vi "GetPathToClass.vi"(8 "error in (no error)":errorcluster, 10 "configuration file path":path=path "") -> (0 "error IO":errorcluster, 2 "PathToClass":path)   [LabVIEW 2014, in "NistBaseClasses.lvlib" / "NISTObject.lvclass"]
uses:
  NISTObject.lvclass
  <vilib>/Utility/config.llb/Read Key (Path).vi
  <vilib>/Utility/config.llb/NI_LVConfig.lvlib
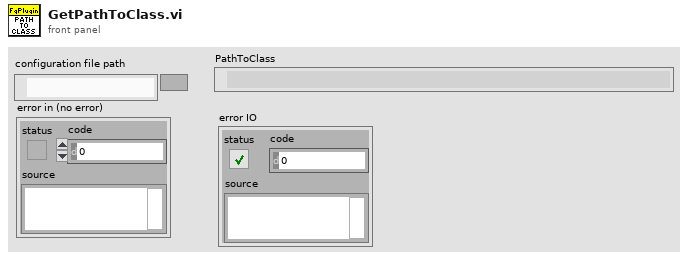
[diagram p1: front panel]
types:
  T1 = typedef "NI_LVConfig.lvlib/Config Data RefNum.ctl" = refnum<k1>
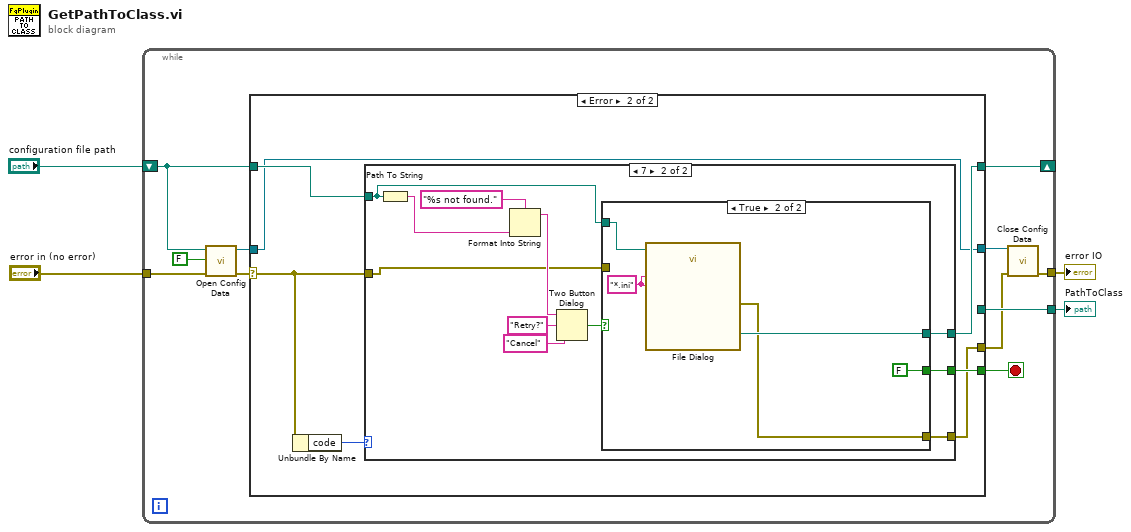
[diagram p0: block diagram]
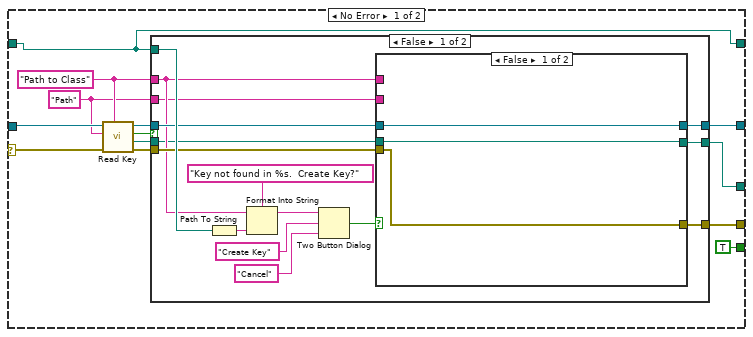
[diagram p2: hidden frame]
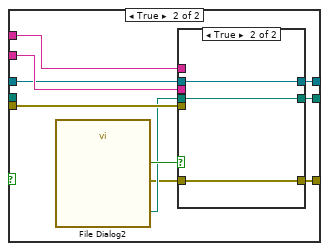
[diagram p3: hidden frame]
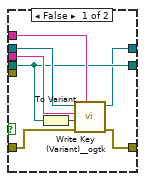
[diagram p4: hidden frame]
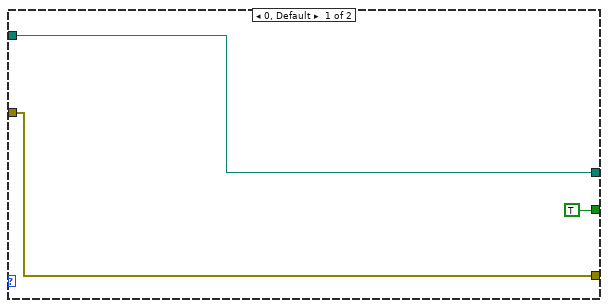
[diagram p6: hidden frame]
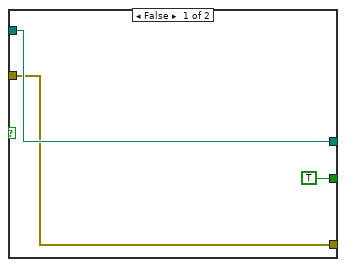
[diagram p7: hidden frame]
diagram:
  n1 = while {
    tunnel: "error in (no error)" -> [w15]
    shift-right: [w11] -> _
    shift-left: "configuration file path" -> [w5]
    tunnel: [w6] -> w2
    tunnel: [w9] -> w1
    stop <- w10 stop-if-true
    n2 = call <vilib>:"Open Config Data.vi"("error in (no error)"=w15, "create file if necessary (T)"=FALSE, "configuration file path"=w5) -> ("error out"=w13:errorcluster, "refnum"=w12:T1)  [unwired: 6 in, 1 out]
    n3 = case shown="Error" w13 {
      selector: w13 -> [w26 w73]
      tunnel: w12 -> [w27 w71]
      tunnel: w5 -> [w20 w76]
      tunnel: [w20 w75] -> w11
      tunnel: [TRUE w74] -> w10
      tunnel: [w17 w72] -> w7
      tunnel: [w18 _] -> w9
      tunnel: [w16 w71] -> w8
      frame No Error {
        w21 = "Path" ("key")
        w24 = "Path to Class" ("section")
        n4 = call-poly <vilib>:"Read Key.vi"("section"=w24, "error in (no error)"=w26, "key"=w21, "refnum"=w27) -> ("error out"=w23:errorcluster, "value"=w19:path, "found?"=w25:bool, "refnum out"=w22:T1)  [unwired: 4 in]
        n5 = case shown="False" w25 {
          tunnel: w24 -> [w34 _]
          tunnel: w23 -> [w36 w69]
          tunnel: w20 -> [w41 _]
          tunnel: w22 -> [w35 w68]
          tunnel: w21 -> [w33 _]
          tunnel: w19 -> [w32 w70]
          tunnel: [w31 w70] -> w18
          tunnel: [w30 w69] -> w17
          tunnel: [w29 w68] -> w16
          frame False {
            n6 = Path To String(path=w41) -> (string=w42:string)
            n7 = Format Into String(format string="Key not found in %s.  Create Key?", initial string=w34, w42) -> (resulting string=w40:string)  [unwired: 1 in, 1 out]
            n8 = Two Button Dialog(message=w40, 1:"Cancel" ("F button name (\"Cancel\")"), 2:"Create Key" ("T button name (\"OK\")")) -> (T button?=w37:bool)
            n9 = case shown="False" w37 {
              tunnel: w36 -> [w45 w54]
              tunnel: w35 -> [w44 w55]
              tunnel: w34 -> [_ w53]
              tunnel: w33 -> [_ w56]
              tunnel: w32 -> [w46 _]
              tunnel: [w46 w50] -> w31
              tunnel: [w45 w49] -> w30
              tunnel: [w44 w47] -> w29
              frame False {
              }
              frame True {
                n10 = call "File Dialog2"() -> ("selected path"=w51:path, "cancelled"=w52:bool, "error out"=w48:errorcluster)  [unwired: 12 in, 1 out]
                n11 = case shown="True" w52 {
                  tunnel: w56 -> [w64 _]
                  tunnel: w55 -> [w63 w65]
                  tunnel: w54 -> [_ _]
                  tunnel: w53 -> [w62 _]
                  tunnel: w51 -> [w60 w67]
                  tunnel: [w60 w67] -> w50
                  tunnel: [w58 w66] -> w49
                  tunnel: w48 -> [w59 w66]
                  tunnel: [w57 w65] -> w47
                  frame False {
                    n12 = To Variant(anything=w60) -> (Variant=w61:variant)
                    n13 = call <userlib>:"Write Key (Variant)__ogtk.vi"("section"=w62, "error in (no error)"=w59, "key-value"=w61, "key (optional)"=w64, "refnum"=w63) -> ("error out"=w58:errorcluster, "refnum out"=w57:T1)  [unwired: 5 in]
                  }
                  frame True {
                  }
                }
              }
            }
          }
          frame True {
          }
        }
      }
      frame Error {
        n14 = Unbundle By Name(w73) -> ("code"=w77:i32)
        n15 = case shown="7" w77 {
          tunnel: w76 -> [w78 w86]
          tunnel: [w78 w85] -> w75
          tunnel: [TRUE w84] -> w74
          tunnel: w73 -> [w79 w83]
          tunnel: [w79 w82] -> w72
          frame 0, Default {
          }
          frame 7 {
            n16 = Path To String(path=w86) -> (string=w81:string)
            n17 = Format Into String(format string="%s not found.", w81) -> (resulting string=w90:string)  [unwired: 2 in, 1 out]
            n18 = Two Button Dialog(message=w90, 1:"Cancel" ("F button name (\"Cancel\")"), 2:"Retry?" ("T button name (\"OK\")")) -> (T button?=w87:bool)
            n19 = case shown="True" w87 {
              tunnel: w86 -> [w93 w95]
              tunnel: [w93 w98] -> w85
              tunnel: [TRUE FALSE] -> w84
              tunnel: w83 -> [w92 _]
              tunnel: [w92 w96] -> w82
              frame False {
              }
              frame True {
                w99 = "*.ini" ("pattern (all files)")
                n20 = call "File Dialog"("start path"=w95, "pattern (all files)"=w99, "pattern label"=w99) -> ("selected path"=w98:path, "error out"=w96:errorcluster)  [unwired: 9 in, 2 out]
              }
            }
          }
        }
      }
    }
    n21 = call <vilib>:"Close Config Data.vi"("error in (no error)"=w7, "refnum"=w8) -> ("error out"=w6:errorcluster)  [unwired: 8 in, 1 out]
  }
  "error IO" <- w2
  "PathToClass" <- w1
